vi "PSVCH_String Replace.vi"(7 "Simple?":bool=TRUE, 8 "Error In (no error)":errorcluster, 9 "ai[] In":string[](array[string]), 10 "Tag[] In":string[](array[string])=["D0", "D1", "D2"], 11 "String In":string="\"D0\"+\"D0\"+\"D1\"+\"D2\"") -> (0 "Error Out":errorcluster, 1 "Tag[] Out":string[](array[string]), 2 "ai[] Out":string[](array[string]), 3 "String Out":string)   [LabVIEW 2016]
panel:
  # "Data In"
  # "Data Out"
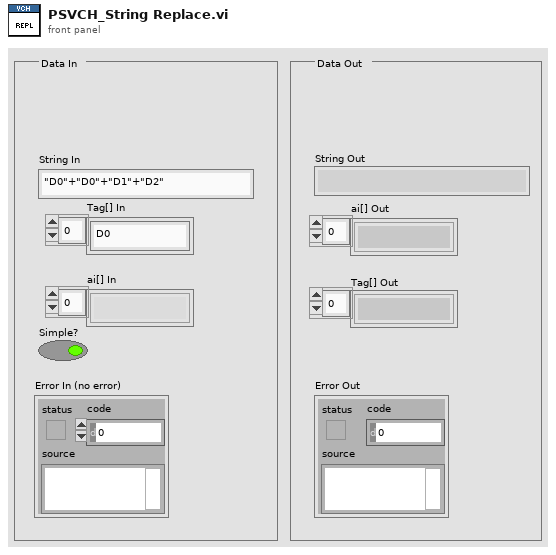
[diagram p1: front panel]
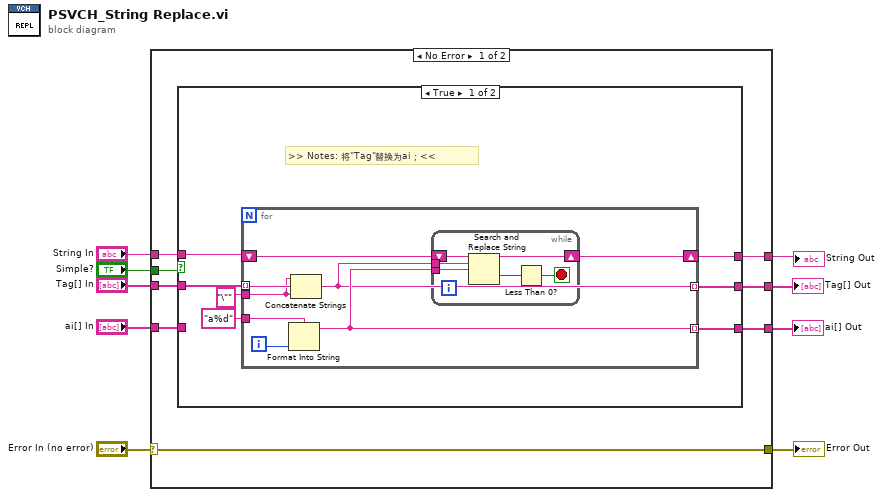
[diagram p0: block diagram]
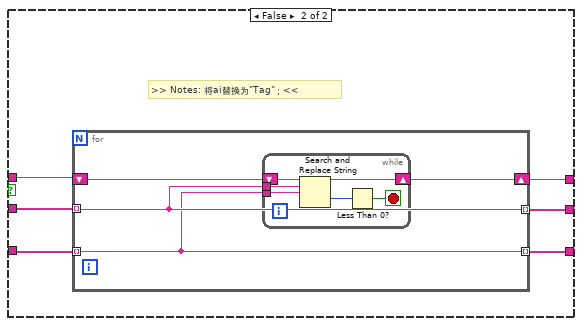
[diagram p2: hidden frame]
diagram:
  n1 = case shown="No Error" "Error In (no error)" {
    selector: "Error In (no error)" -> [w10 w55]
    tunnel: "String In" -> [w17 _]
    tunnel: "Tag[] In" -> [w16 _]
    tunnel: [w15 _] -> w7
    tunnel: [w14 _] -> w6
    tunnel: [w13 _] -> w5
    tunnel: "ai[] In" -> [w12 _]
    tunnel: "Simple?" -> [w11 _]
    tunnel: [w10 w55] -> w1
    frame No Error {
      n2 = case shown="True" w11 {
        tunnel: w17 -> [w24 w44]
        tunnel: w16 -> [w23 w43]
        tunnel: [w20 w42] -> w15
        tunnel: [w19 w41] -> w14
        tunnel: [w18 w40] -> w13
        tunnel: w12 -> [_ w39]
        frame True {
          # ">> Notes: 将\"Tag\"替换为ai；<<"
          n3 = for {
            tunnel: w23 -> [w32] mode=indexing
            tunnel: "\"" ("字符串") -> [w30]
            tunnel: "a%d" ("字符串") -> [w29]
            shift-right: [w27] -> w20
            shift-left: w24 -> [w31]
            tunnel: [w26] -> w19 mode=indexing
            tunnel: [w25] -> w18 mode=indexing
            i -> [w28]
            n4 = Format Into String(format string=w29, w28) -> (resulting string=w26:string)  [unwired: 2 in, 1 out]
            n5 = Concatenate Strings(w30, w32, w30) -> (w25:string)
            n6 = while {
              tunnel: w26 -> [w36]
              tunnel: w25 -> [w35]
              shift-right: [w37] -> w27
              shift-left: w31 -> [w38]
              stop <- w33 stop-if-true
              n7 = Search and Replace String(input string=w38, search string=w35, replace string=w36) -> (result string=w37:string, offset past replacement=w34:i32)  [unwired: 5 in, 2 out]
              n8 = Less Than 0?(x=w34) -> (x < 0?=w33:bool)
            }
          }
        }
        frame False {
          # ">> Notes: 将ai替换为\"Tag\"；<<"
          n9 = for {
            tunnel: w43 -> [w46] mode=indexing
            shift-right: [w47] -> w42
            shift-left: w44 -> [w48]
            tunnel: [w45] -> w41 mode=indexing
            tunnel: [w46] -> w40 mode=indexing
            tunnel: w39 -> [w45] mode=indexing
            n10 = while {
              tunnel: w45 -> [w52]
              tunnel: w46 -> [w51]
              shift-right: [w53] -> w47
              shift-left: w48 -> [w54]
              stop <- w49 stop-if-true
              n11 = Search and Replace String(input string=w54, search string=w51, replace string=w52) -> (result string=w53:string, offset past replacement=w50:i32)  [unwired: 5 in, 2 out]
              n12 = Less Than 0?(x=w50) -> (x < 0?=w49:bool)
            }
          }
        }
      }
    }
    frame Error {
    }
  }
  "String Out" <- w7
  "ai[] Out" <- w6
  "Tag[] Out" <- w5
  "Error Out" <- w1
